vi "Handle Message.vi"(8 "error in":errorcluster, 10 "Message":T1, 11 "Vision Server in":refnum<class "Vision Server.lvclass">) -> (0 "error out":errorcluster, 3 "Vision Server out":refnum<class "Vision Server.lvclass">)   [LabVIEW 2016, in "Vision Server.lvclass"]
uses:
  Vision Server.lvclass
  typedef/Message Type.ctl
  Vision Server.lvclass/Vision Server.ctl
  typedef/Target Message JSON.ctl
  typedef/Target Vector.ctl
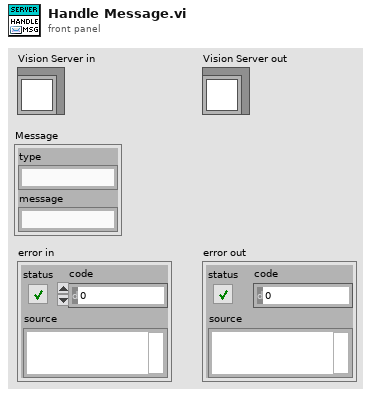
[diagram p1: front panel]
types:
  T1 = typedef "Vision Server.lvclass/Message Type.ctl" = cluster{"type":string, "message":string}
  T2 = typedef "Vision Server.lvclass/Target Message JSON.ctl" = cluster{"capturedAgoMs":i32, "targets":T3[]}
  T3 = typedef "Vision Server.lvclass/Target Vector.ctl" = cluster{"y":dbl, "z":dbl}
  T4 = typedef "Vision Server.lvclass/Target Listener Queue.ctl" = refnum<queue>
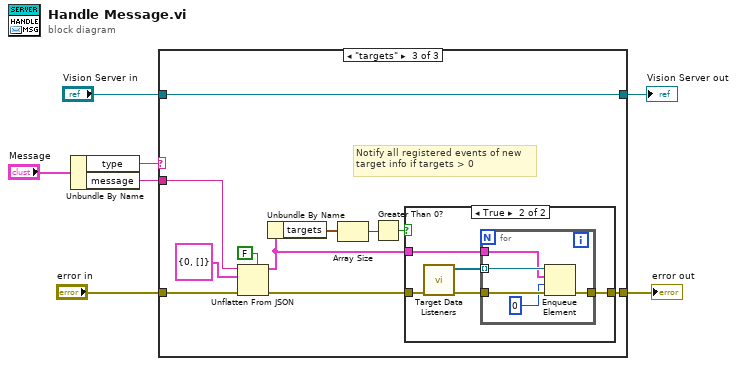
[diagram p0: block diagram]
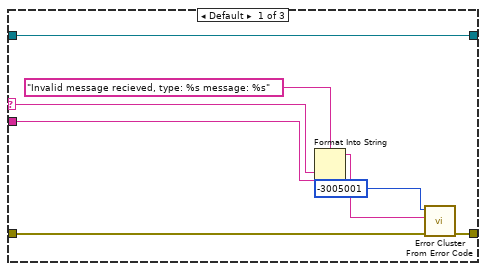
[diagram p2: hidden frame]
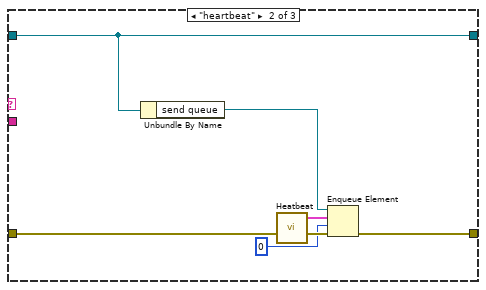
[diagram p3: hidden frame]
diagram:
  n1 = Unbundle By Name("Message") -> ("type"=w2:string, "message"=w1:string)
  n2 = case shown="\"targets\"" w2 {
    selector: w2 -> [w12 _ _]
    tunnel: "error in" -> [w15 w19 w28]
    tunnel: [w13 w18 w26] -> w5
    tunnel: "Vision Server in" -> [w14 w21 w32]
    tunnel: [w14 w21 w32] -> w7
    tunnel: w1 -> [w11 _ w31]
    frame Default {
      n3 = Format Into String(format string="Invalid message recieved, type: %s message: %s" ("error message (\"\")"), w12, w11) -> (resulting string=w8:string)  [unwired: 2 in, 1 out]
      n4 = call <vilib>:"Error Cluster From Error Code.vi"("error in (no error)"=w15, "error message (\"\")"=w8, "error code (0)"=-3005001) -> ("error out"=w13:errorcluster)  [unwired: 6 in]
    }
    frame "heartbeat" {
      n5 = Unbundle By Name(w21) -> ("send queue"=w20:refnum<queue>)
      n6 = call "Heatbeat.vi"() -> ("camera mode vision"=w17:T1)  [unwired: 2 in]
      n7 = Enqueue Element(queue=w20, element=w17, timeout in ms (-1)=0, error in (no error)=w19) -> (error out=w18:errorcluster)  [unwired: 2 out]
    }
    frame "targets" {
      # "Notify all registered events of new\ntarget info if targets > 0"
      n8 = Unflatten From JSON(enable LabVIEW extensions? (T)=FALSE, JSON string=w31, type and defaults=T2 {"capturedAgoMs"=0, "targets"=[]}, error in (no error)=w28) -> (value=w25:T2, error out=w27:errorcluster)  [unwired: 3 in]
      n9 = Unbundle By Name(w25) -> ("targets"=w24:T3[])
      n10 = Array Size(array=w24) -> (size(s)=w22:i32)
      n11 = Greater Than 0?(x=w22) -> (x > 0?=w23:bool)
      n12 = case shown="True" w23 {
        tunnel: w27 -> [w33 w34]
        tunnel: w25 -> [_ w36]
        tunnel: [w33 w35] -> w26
        frame False {
          # "0 targets found"
        }
        frame True {
          n13 = call "Target Data Listeners.vi"("error in"=w34) -> ("error out"=w38:errorcluster, "Listeners"=w37:T4[])  [unwired: 9 in]
          n14 = for {
            tunnel: w38 -> [w42]
            tunnel: w37 -> [w43] mode=indexing
            tunnel: w36 -> [w41]
            tunnel: [w39] -> w35
            n15 = Enqueue Element(queue=w43, element=w41, timeout in ms (-1)=0, error in (no error)=w42) -> (error out=w39:errorcluster)  [unwired: 2 out]
          }
        }
      }
    }
  }
  "Vision Server out" <- w7
  "error out" <- w5
